vi "New_FPGA_Hex_Gen.vi"(9 "Laser(V)":dbl[](array[numeric]), 11 "Chirp Parameters":T19) -> (1 "HEX Array":string[](array[string]), 3 "Interrupted":bool)   [LabVIEW 2017]
uses:
  Controls/Frequency Record.ctl
  Global Variables/General Globals.vi
  Typedefs/HW config states enum.ctl
  Controls/Pockels_Galvo_Params.ctl
  Typedefs/Chirp_ABCD.ctl
  Typedefs/XY Stage config cluster.ctl
  Typedefs/Cam VidRec HW config setup cluster.ctl
  Typedefs/Control Sys HW config cluster.ctl
  <vilib>/userdefined/High Color/nirio_resource_hc.ctl
  Typedefs/FPGA input type AC-DC.ctl
  Typedefs/DAQmx physical channels cluster.ctl
  Typedefs/Encoder config cluster.ctl
  Typedefs/Z Stage config cluster.ctl
  Typedefs/Laser 1 config cluster.ctl
  Typedefs/PreChirper 1 config cluster.ctl
  Typedefs/Laser Power Control HW config.ctl
  Typedefs/Triggers HW config.ctl
  Typedefs/Hardware Configuration settings.ctl
  RIG-SPECIFIC FILES/FPGA Refs/FPGA Ref.ctl
  Typedefs/DAQ FPGA system config.ctl
  Typedefs/CTRL system config.ctl
  Typedefs/System Configuration.ctl
  Typedefs/DAQ FPGA HW config cluster.ctl
panel:
  in  "System Config":T1={"Laser wavelength (nm)"=920.0, "DAQ FPGA System"={"Clock Freq (MHz) "=200.0, "Samples Wait after Trigger"=5080, "AOD fill"=4900, "StartupDelay"=0, "Slip Cycle (clock cycles)"=600000, "Add Cycle"=TRUE}, "Control system"={"AOD 1 Amplitude"=0, "AOD 2 Amplitude"=0, "AOD 3 Amplitude"=0, "AOD 4 Amplitude"=0, "AOD 5 Amplitude"=0, "AOD 6 Amplitude"=0, "T0 (ns)"=0.0, "Ta (ns)"=0.0, "Data Time Interval (ns)"=0.0, "Ctrl FPGA Clock (MHz)"=240.0}} {"Control system"."Ctrl FPGA Clock (MHz)" min=80.0 max=500.0 step=1.0; "Control system"."Data Time Interval (ns)" min=0.0 max=2048.0 step=1.0; "Control system"."Ta (ns)" min=0.0 max=2048.0 step=1.0; "Control system"."T0 (ns)" min=0.0 max=2048.0 step=1.0; "Control system"."AOD 6 Amplitude" min=0 max=2048 step=1; "Control system"."AOD 5 Amplitude" min=0 max=2048 step=1; "Control system"."AOD 4 Amplitude" min=0 max=2048 step=1; "Control system"."AOD 3 Amplitude" min=0 max=2048 step=1; "Control system"."AOD 2 Amplitude" min=0 max=2048 step=1; "Control system"."AOD 1 Amplitude" min=0 max=2048 step=1; "Laser wavelength (nm)" min=800.0 max=1080.0 step=1.0}
  in  "Hardware Config":T4={"Dev. PC"=FALSE, "Swap XY on stage"=FALSE, "No of AOD"=0, "Computer MAC address"="", "Externalise Triggers"=FALSE, "Trigger HW config"={"Available Device List"=0, "Device Address"=""}, "DAQmx Chan"={"Pockels AO"="", "Hard shutter AO"="", "PMT AOs"="", "Galvo AOs"="", "Power meter AI"=""}, "XY stage available"=FALSE, "XY Stage"={"COM port"="", "Baudrate"=0, "Type"=""}, "Z stage available"=FALSE, "Z Stage config cluster"={"COM port"="COM7", "Baudrate"=0, "Type"=""}, "Encoder available"=FALSE, "Encoder"={"IP address"="224.0.1.103", "Port"=7000, "Wheel radius (cm)"=16.0, "Encoder Trigger"=""}, "VidRec available"=FALSE, "Cam VidRec"={"DO flag-Video record"="", "DO flag-Trial start"=""}, "Laser Power Control HW config"={"Laser Power Control"="", "Laser Power Modulation Control"=enum."NI"}, "Laser 1 available"=FALSE, "Laser 1 config cluster"={"COM port"="COM7", "Baud Rate"=0, "Type"=""}, "Prechirper 1 available"=FALSE, "Prechirper 1 config cluster"={"Type"="", "Baud Rate"=0, "COM port"="COM7"}, "Control system.FPGA available?"=FALSE, "Control Sys. HW config"={"Control system.FPGA Type"=enum."Virtex 5", "Control system.Network adapter name"="", "Control system.MAC address"="", "Control system.Ethernet Port"=0, "Control system.Ethernet Port Opened"=FALSE}, "DAQ FPGA HW Config"={"FGPA Ref"=refnum, "Target"="RIO0", "input card type"=enum."AC Card"}} {"Encoder"."Wheel radius (cm)" format="%#_13g"}
  out "difftime - aodcontrol delay":dbl
  out "diff time":dbl
  in  "frontpanel":bool
  out "Loop index":i32
  # "RE-ENTRANT"
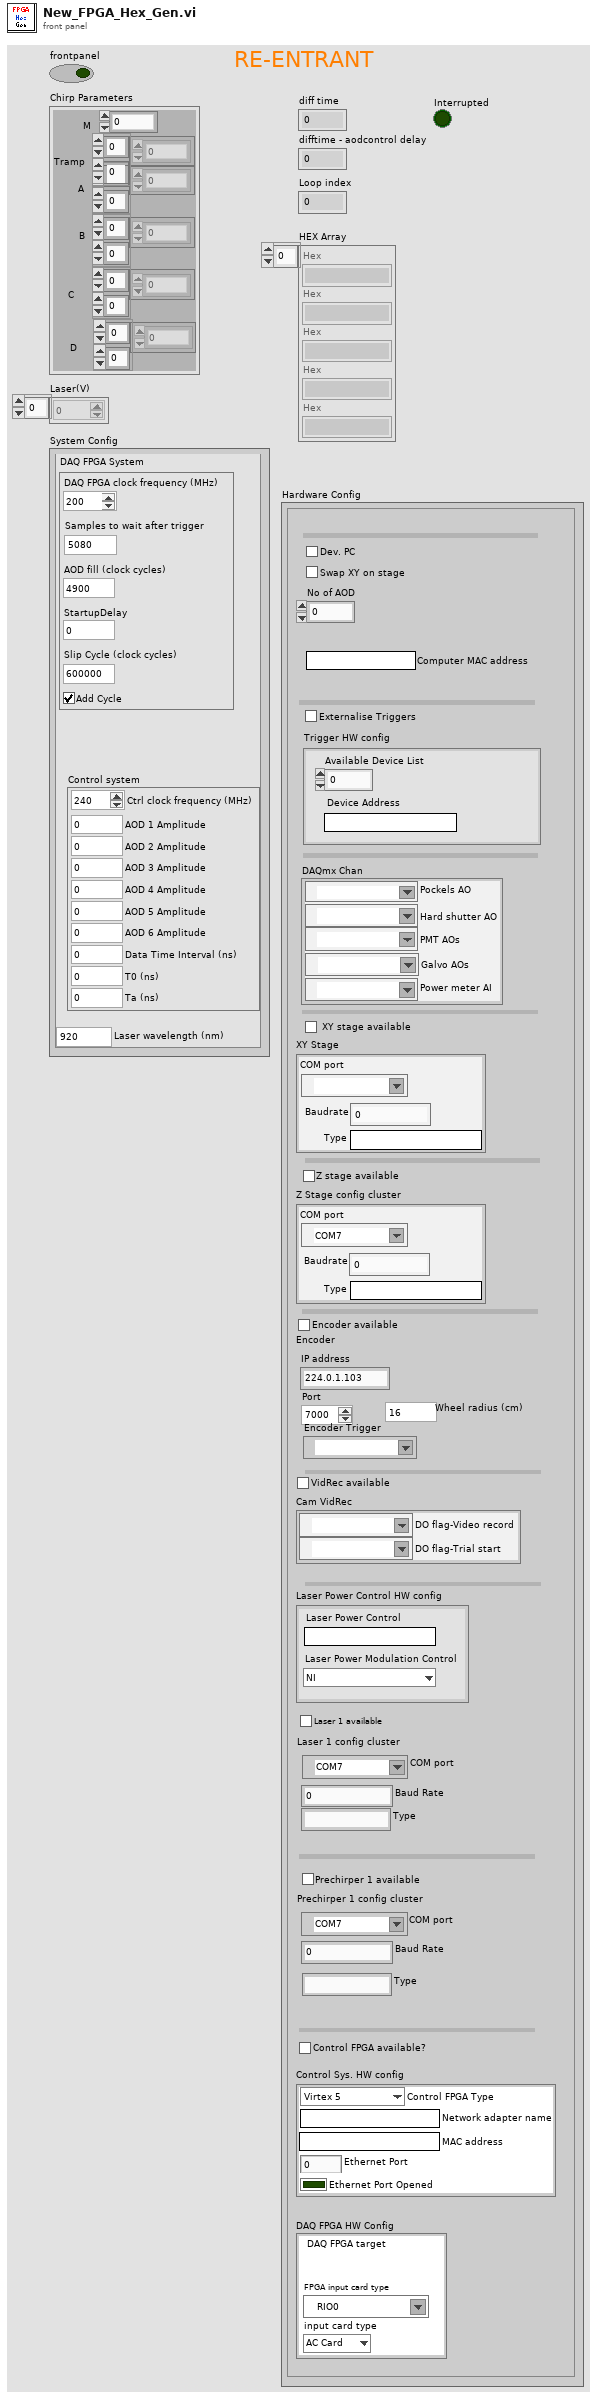
[diagram p1: front panel]
types:
  T1 = typedef "System Configuration.ctl" = cluster{"Laser wavelength (nm)":dbl, "DAQ FPGA System":T2, "Control system":T3}
  T2 = typedef "DAQ FPGA system config.ctl" = cluster{"Clock Freq (MHz) ":dbl, "Samples Wait after Trigger":u16, "AOD fill":u16, "StartupDelay":i32, "Slip Cycle (clock cycles)":u32, "Add Cycle":bool}
  T3 = typedef "CTRL system config.ctl" = cluster{"AOD 1 Amplitude":i16, "AOD 2 Amplitude":i16, "AOD 3 Amplitude":i16, "AOD 4 Amplitude":i16, "AOD 5 Amplitude":i16, "AOD 6 Amplitude":i16, "T0 (ns)":dbl, "Ta (ns)":dbl, "Data Time Interval (ns)":dbl, "Ctrl FPGA Clock (MHz)":dbl}
  T4 = typedef "Hardware Configuration settings.ctl" = cluster{"Dev. PC":bool, "Swap XY on stage":bool, "No of AOD":u8, "Computer MAC address":string, "Externalise Triggers":bool, "Trigger HW config":T5, "DAQmx Chan":T6, "XY stage available":bool, "XY Stage":T7, "Z stage available":bool, "Z Stage config cluster":T8, "Encoder available":bool, "Encoder":T9, "VidRec available":bool, "Cam VidRec":T10, "Laser Power Control HW config":T11, "Laser 1 available":bool, "Laser 1 config cluster":T12, "Prechirper 1 available":bool, "Prechirper 1 config cluster":T13, "Control system.FPGA available?":bool, "Control Sys. HW config":T14, "DAQ FPGA HW Config":T15}
  T5 = typedef "Triggers HW config.ctl" = cluster{"Available Device List":i32, "Device Address":string}
  T6 = typedef "DAQmx physical channels cluster.ctl" = cluster{"Pockels AO":tag, "Hard shutter AO":tag, "PMT AOs":tag, "Galvo AOs":tag, "Power meter AI":tag}
  T7 = typedef "XY Stage config cluster.ctl" = cluster{"COM port":refnum<visa-resource-name>, "Baudrate":i32, "Type":string}
  T8 = typedef "Z Stage config cluster.ctl" = cluster{"COM port":refnum<visa-resource-name>, "Baudrate":i32, "Type":string}
  T9 = typedef "Encoder config cluster.ctl" = cluster{"IP address":string, "Port":u16, "Wheel radius (cm)":dbl, "Encoder Trigger":tag}
  T10 = typedef "Cam VidRec HW config setup cluster.ctl" = cluster{"DO flag-Video record":tag, "DO flag-Trial start":tag}
  T11 = typedef "Laser Power Control HW config.ctl" = cluster{"Laser Power Control":string, "Laser Power Modulation Control":enum16{"NI", "FPGA"}}
  T12 = typedef "Laser 1 config cluster.ctl" = cluster{"COM port":refnum<visa-resource-name>, "Baud Rate":i32, "Type":string}
  T13 = typedef "PreChirper 1 config cluster.ctl" = cluster{"Type":string, "Baud Rate":i32, "COM port":refnum<visa-resource-name>}
  T14 = typedef "Control Sys HW config cluster.ctl" = cluster{"Control system.FPGA Type":enum16{"Virtex 5", "Virtex 7"}, "Control system.Network adapter name":string, "Control system.MAC address":string, "Control system.Ethernet Port":u32, "Control system.Ethernet Port Opened":bool}
  T15 = typedef "DAQ FPGA HW config cluster.ctl" = cluster{"FGPA Ref":T16, "Target":T17, "input card type":T18}
  T16 = typedef "FPGA Ref.ctl" = refnum<k20>
  T17 = typedef "nirio_resource_hc.ctl" = tag
  T18 = typedef "FPGA input type AC-DC.ctl" = enum16{"AC Card", "DC Card"}
  T19 = typedef "Chirp_ABCD.ctl" = cluster{"M ":dbl, "Tramp":dbl[][], "A":dbl[][], "B":dbl[][], "C":dbl[][], "D":dbl[][]}
  T20 = typedef "Pockels_Galvo_Params.ctl" = cluster{"A":dbl[], "Pockels Level":dbl[], "X Galvo":dbl[], "Y Galvo":dbl[], "AOD Fill Cycles":dbl[]}
  T21 = typedef "Frequency Record.ctl" = cluster{"Phi":dbl[], "A":dbl[], "B":dbl[], "C":dbl[], "D":dbl[], "E":dbl[], "Tstart":dbl[], "Tframe":dbl[]}
  T22 = typedef "HW config states enum.ctl" = enum16{"Load from file", "Save to file", "Write all", "Read all", "Write XY stage settings", "Write DAQ FPGA settings", "Write Control FPGA settings", "Write Phys Channels", "Write System Config", "Write HW Config", "Save System Config", "Save HW Config", "Clear", "Compare from file"}
  T23 = typedef "Hardware Configuration settings.ctl" = cluster{"Dev. PC":bool, "Swap XY on stage":bool, "No of AOD":u8, "MC Supported":bool, "Axial MC":bool, "Computer MAC address":string, "Externalise Triggers":bool, "Trigger HW config":T5, "DAQmx Chan":T6, "XY stage available":bool, "XY Stage":T7, "Z stage available":bool, "Z Stage config cluster":T8, "Encoder available":bool, "Encoder":T9, "VidRec available":bool, "Cam VidRec":T10, "Laser Power Control HW config":T11, "Laser 1 available":bool, "Laser 1 config cluster":T12, "Prechirper 1 available":bool, "Prechirper 1 config cluster":T13, "Control system.FPGA available?":bool, "Control Sys. HW config":T14, "DAQ FPGA HW Config":T15}
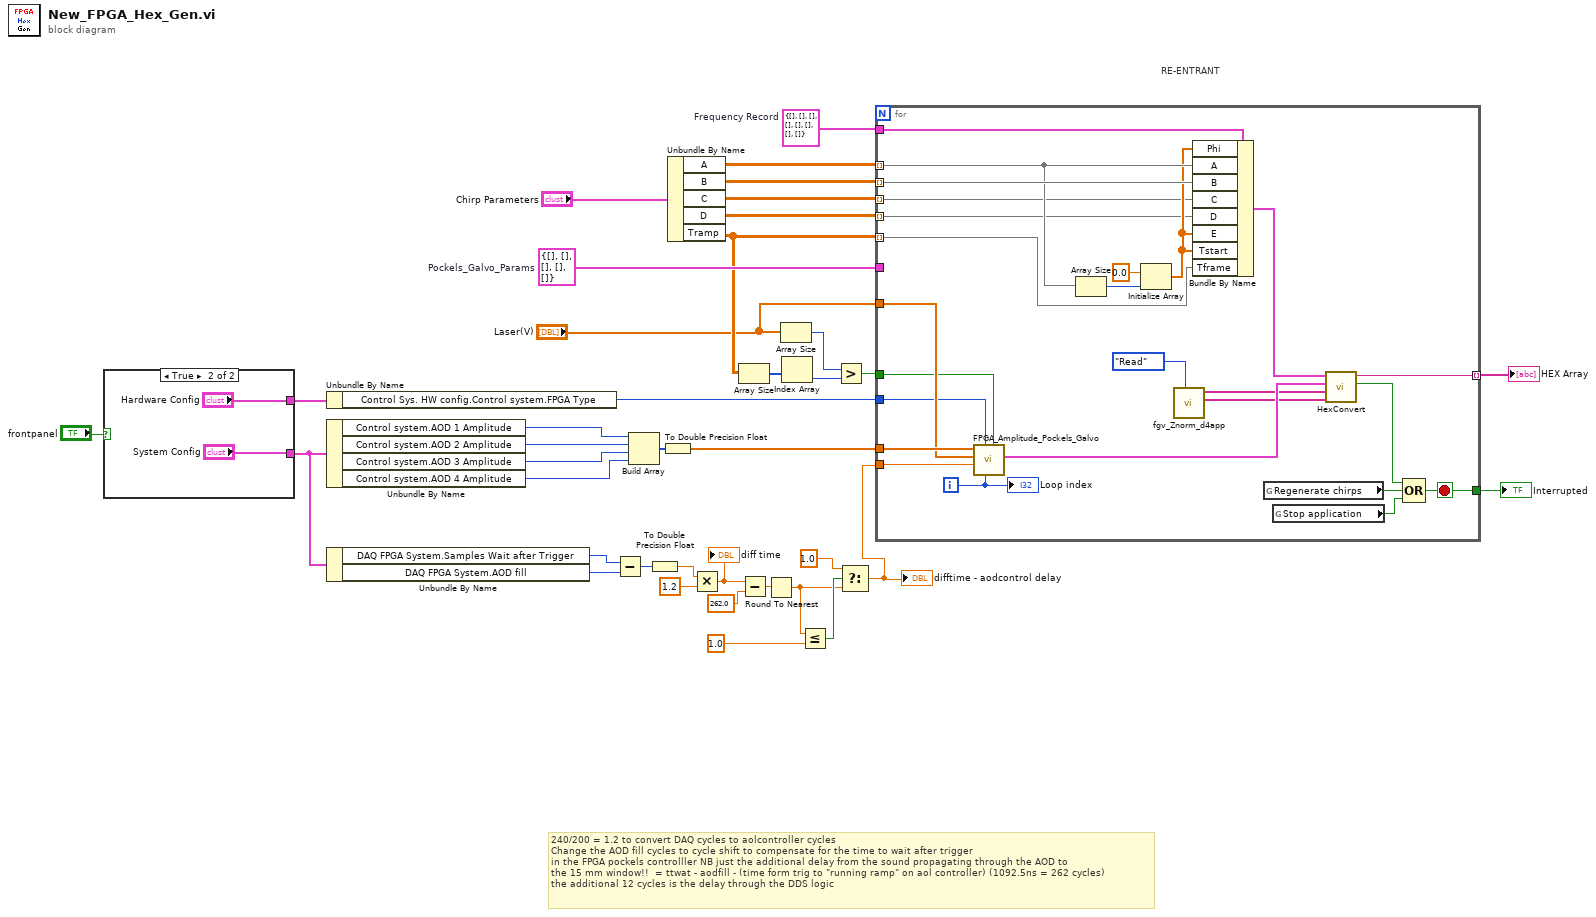
[diagram p0: block diagram]
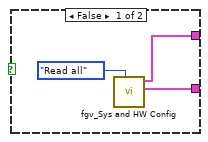
[diagram p2: hidden frame]
diagram:
  w24 = T20 {"A"=[], "Pockels Level"=[], "X Galvo"=[], "Y Galvo"=[], "AOD Fill Cycles"=[]}  # Pockels_Galvo_Params
  w38 = T21 {"Phi"=[], "A"=[], "B"=[], "C"=[], "D"=[], "E"=[], "Tstart"=[], "Tframe"=[]}  # Frequency Record
  # "240/200 = 1.2 to convert DAQ cycles to aolcontroller cycles\nChange the AOD fill cycles to cycle shift to compensate for the time to wait after trigger\nin the FPGA pockels controlller NB just the additional delay from the sound propagating through the AOD to\nthe 15 mm window!!  = ttwat - aodfill - (time form trig to \"running ramp\" on aol controller) (1092.5ns = 262 cycles)\nthe additional 12 cycles is the delay through the DDS logic"
  # "RE-ENTRANT"
  n1 = case shown="True" "frontpanel" {
    tunnel: [w40 "System Config"] -> w9
    tunnel: [w39 "Hardware Config"] -> w8
    frame False {
      n2 = call "fgv_Sys and HW Config.vi"("Function"=HW_config_states_enum."Read all") -> ("System Config OUT"=w40:T1, "Hardware Configuration OUT"=w39:T23)  [unwired: 8 in, 1 out]
    }
    frame True {
    }
  }
  n3 = Unbundle By Name(w8) -> ("Control Sys. HW config.Control system.FPGA Type"=w7:enum16{"Virtex 5", "Virtex 7"})
  n4 = Unbundle By Name(w9) -> ("Control system.AOD 1 Amplitude"=w35:i16, "Control system.AOD 2 Amplitude"=w34:i16, "Control system.AOD 3 Amplitude"=w33:i16, "Control system.AOD 4 Amplitude"=w32:i16)
  n5 = Unbundle By Name(w9) -> ("DAQ FPGA System.Samples Wait after Trigger"=w18:u16, "DAQ FPGA System.AOD fill"=w17:u16)
  n6 = Subtract(x=w18, y=w17) -> (x-y=w16:u16)
  n7 = Build Array(w35, w34, w33, w32) -> (w30:i16[])
  n8 = To Double Precision Float(number=w16) -> (double precision float=w15:dbl)
  n9 = To Double Precision Float(number=w30) -> (double precision float=w26:dbl[])
  n10 = Unbundle By Name("Chirp Parameters") -> ("A"=w31:dbl[][], "B"=w6:dbl[][], "C"=w29:dbl[][], "D"=w28:dbl[][], "Tramp"=w23:dbl[][])
  n11 = Multiply(x=w15, y=1.2) -> (x*y=w13:dbl)
  "diff time" <- w13
  n12 = Array Size(array=w23) -> (size(s)=w22:i32[])
  n13 = Subtract(x=w13, y=262.0) -> (x-y=w11:dbl)
  n14 = Round To Nearest(number=w11) -> (nearest integer value=w2:dbl)
  n15 = Array Size(array="Laser(V)") -> (size(s)=w20:i32)
  n16 = Index Array(array=w22) -> (element=w21:i32)  [unwired: 1 in]
  n17 = Less Or Equal?(x=w2, y=1.0) -> (x <= y?=w4:bool)
  n18 = Greater?(x=w20, y=w21) -> (0:w19:bool)
  n19 = Select(t=1.0, s=w4, f=w2) -> (s? t:f=w1:dbl)
  "difftime - aodcontrol delay" <- w1
  n20 = for {
    tunnel: w31 -> [w63] mode=indexing
    tunnel: w38 -> [w65]
    tunnel: w24 -> [_]
    tunnel: w26 -> [w52]
    tunnel: w29 -> [w55] mode=indexing
    tunnel: w6 -> [w64] mode=indexing
    tunnel: w28 -> [w54] mode=indexing
    tunnel: [w61] -> w36 mode=indexing
    tunnel: [w60] -> w27
    tunnel: w23 -> [w57] mode=indexing
    tunnel: w1 -> [w50]
    tunnel: "Laser(V)" -> [w51]
    tunnel: w19 -> [w47]
    tunnel: w7 -> [w48]
    i -> [w49]
    stop <- w60 stop-if-true
    n21 = call "FPGA_Amplitude_Pockels_Galvo.vi"("Live(F)/Functional(T)"=w47, "Chirp index"=w49, "FPGA Type"=w48, "difftime - aodcontrol delay"=w50, "Laser(V) - Vertex 7 Only"=w51, "Amplitude"=w52) -> ("Pockels_Galvo_Params"=w53:T20)  [unwired: 5 in]
    n22 = Array Size(array=w63) -> (size(s)=w66:i32)
    n23 = Initialize Array(0.0 ("element"), w66) -> (w56:dbl[])
    n24 = call "fgv_Znorm_d4app.vi"("Function"=enum16{"Idle", "Write", "Read"}."Read") -> ("E Field"=w44:string[], "Phase Field"=w45:string[])  [unwired: 8 in, 1 out]
    n25 = Bundle By Name(cluster=w65, "Phi"=w56, "A"=w63, "B"=w64, "C"=w55, "D"=w54, "E"=w56, "Tstart"=w56, "Tframe"=w57) -> (w62:T21)
    n26 = global read "General Globals.vi" "Regenerate chirps"() -> (w60:bool)
    n27 = global read "General Globals.vi" "Stop application"() -> (w58:bool)
    n28 = call "HexConvert.vi"("E Field"=w44, "Phase Field"=w45, "Pockels_Galvo_Params"=w53, "Frequency Record"=w62) -> ("Interrupted"=w59:bool, "Hex"=w61:string)  [unwired: 6 in]
    n29 = Compound Arithmetic op=OR(w59, w60, w58) -> ()  [unwired: 1 out]
    "Loop index" <- w49
  }
  "HEX Array" <- w36
  "Interrupted" <- w27
